vi "Init.vi"(8 "error in (no error)":errorcluster, 11 "Vehicle in":refnum<class "Vehicle.lvclass">) -> (0 "error out":errorcluster, 3 "Vehicle out":refnum<class "Vehicle.lvclass">)   [LabVIEW 2019, in "Vehicle.lvclass"]
uses:
  Vehicle.lvclass
  Vehicle.lvclass/Vehicle.ctl
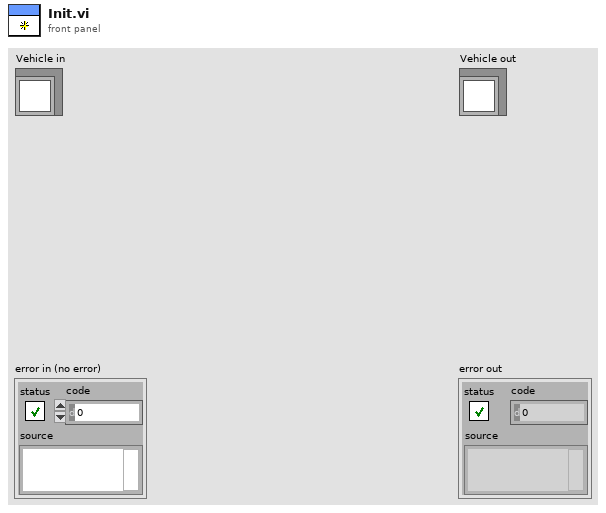
[diagram p1: front panel]
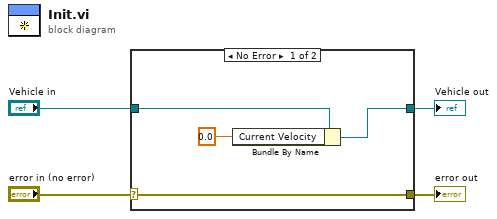
[diagram p0: block diagram]
diagram:
  n1 = case shown="No Error" "error in (no error)" {
    selector: "error in (no error)" -> [w8 w10]
    tunnel: [w8 w10] -> w3
    tunnel: [w5 w9] -> w1
    tunnel: "Vehicle in" -> [w7 w9]
    frame No Error {
      n2 = Bundle By Name(cluster=w7, "Current Velocity"=0.0) -> (w5:refnum<class "Vehicle.lvclass">)
    }
    frame Error {
    }
  }
  "error out" <- w3
  "Vehicle out" <- w1
